vi "Tag.value_lua.vi"(5 "LuaVIEW reference":T1) -> (15 "error out":errorcluster)   [LabVIEW 2012]
doc: "Returns the current value of a tag. This equals the value of the last point written to the tag's in-memory buffer. On initialisation, the datalogger rebuffers the last point which is therefore guaranteed to be available.\nParameters:\nobj:tag\nResults:\nnum:value, value of last written point.\nErrors:\nDead or invalid tag object.\nData logger not initialized."
uses:
  luaview/typedefs/t_LuaVIEW Reference.ctl
  typedefs/t_DataLog Tag Buffers Methods.ctl
  luaview/subvis/private/LuaVIEW Pull (object).vi
  luaview/subvis/private/LuaVIEW Push (number).vi
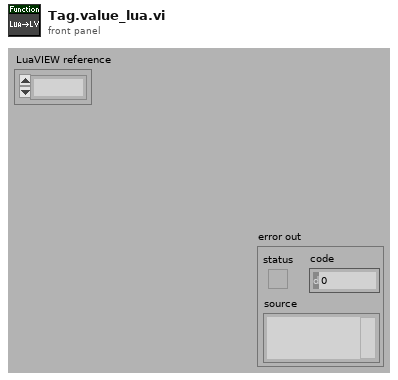
[diagram p1: front panel]
types:
  T1 = typedef "t_LuaVIEW Reference.ctl" = refnum<k1>
  T2 = typedef "t_DataLog Tag Buffers Methods.ctl" = enum16{"initialize", "inert", "write", "read", "read oldest", "read last", "cleanup"}
  T3 = typedef "t_DataLog Point.ctl" = cluster{"time":dbl, "value":dbl}
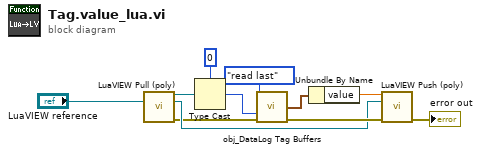
[diagram p0: block diagram]
diagram:
  n1 = call-poly "LuaVIEW Pull (poly).vi"("LuaVIEW reference in"="LuaVIEW reference") -> ("object refnum"=w4:refnum<vi>, "LuaVIEW reference out"=w7:T1, "error out"=w6:errorcluster)  [unwired: 11 in, 1 out]
  n2 = Type Cast(type=0 ("read index in"), x=w4) -> (*(type *) &x=w2:i32)
  n3 = call "obj_DataLog Tag Buffers.vi"("method"=t_DataLog_Tag_Buffers_Methods."read last", "tag index"=w2, "error in (no error)"=w6) -> ("point out"=w10:T3, "error out"=w8:errorcluster)  [unwired: 8 in, 3 out]
  n4 = Unbundle By Name(w10) -> ("value"=w9:dbl)
  n5 = call-poly "LuaVIEW Push (poly).vi"("number"=w9, "LuaVIEW reference in"=w7, "error in (no error)"=w8) -> ("error out"=→"error out":errorcluster)  [unwired: 11 in, 1 out]
